vi "CheckInputFrequency.vi"(4 "Connection ID TB":refnum<k5>, 5 "ERROR IN":errorcluster, 6 "IP ADDRESS":string="192.168.0.2", 7 "TS1 / TS2":bool, 8 "Connection ID CC":refnum<k5>) -> (0 "ERROR OUT":errorcluster, 1 "Success":bool=TRUE, 3 "String":string)   [LabVIEW 2013]
panel:
  out "PROGRESS":i32(slide) scale=0.0..12.0
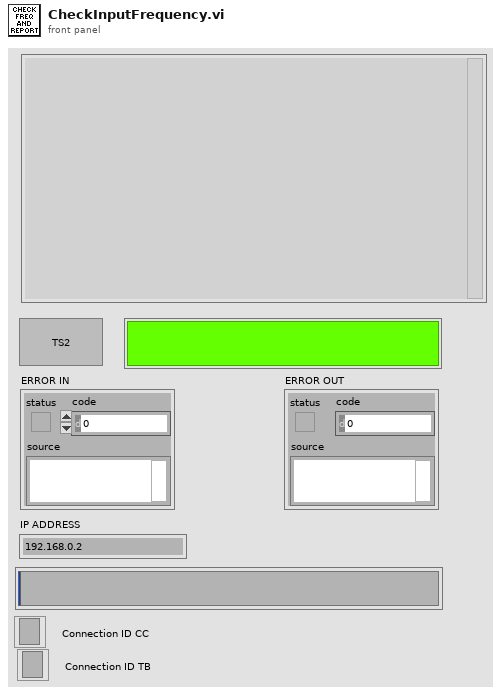
[diagram p1: front panel]
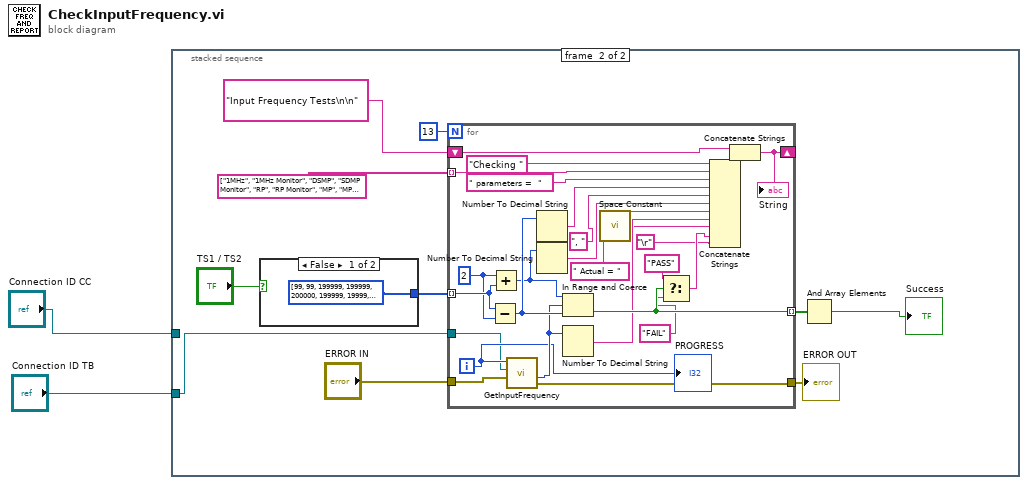
[diagram p0: block diagram]
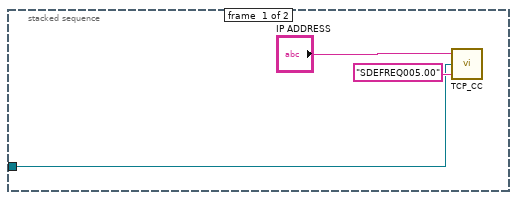
[diagram p2: hidden frame]
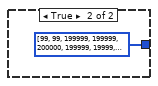
[diagram p3: hidden frame]
diagram:
  n1 = stacked-sequence {
    tunnel: "Connection ID CC" -> [w3 _]
    tunnel: "Connection ID TB" -> [_ w6]
    frame #0 {
      n2 = call "TCP_CC.vi"("COMMAND"="SDEFREQ005.00", "connection ID"=w3, "IP ADDRESS"="IP ADDRESS") -> ()  [unwired: 3 out]
    }
    frame #1 {
      n3 = case shown="False" "TS1 / TS2" {
        tunnel: [u32[] [99, 99, 199999, 199999, 200000, 199999, 19999, 19999, 1199999, 99999, 199999, 199999, 199999] ("Array") u32[] [99, 99, 199999, 199999, 200000, 199999, 19999, 19999, 1199999, 99999, 199999, 199999, 199999] ("Array")] -> w12
        frame False {
        }
        frame True {
        }
      }
      n4 = for {
        N: 13 -> [_]
        tunnel: "ERROR IN" -> [w43]
        tunnel: [w42] -> w14
        tunnel: w12 -> [w20] mode=indexing
        tunnel: [w37] -> w8 mode=indexing
        tunnel: string[] ["1MHz", "1MHz Monitor", "DSMP", "SDMP Monitor", "RP", "RP Monitor", "MP", "MP Monitor", "EEP 1.2", "EEP Monitor", "SMP DIFF", "SMP Monitor", "SMP OC"] -> [w31] mode=indexing
        shift-right: [w21] -> _
        shift-left: "Input Frequency Tests\n\n" -> [w33]
        tunnel: w6 -> [w18]
        i -> [w22]
        w19 = u32 2 ("x")
        n5 = Subtract(x=w20, y=w19) -> (x-y=w41:u32)
        n6 = Add(x=w19, y=w20) -> (x+y=w40:u32)
        n7 = call "GetInputFrequency.vi"("Signal Type Select"=w22, "Connection ID IN"=w18, "ERROR IN"=w43) -> ("DECIMAL"=w38:u32, "ERROR OUT"=w42:errorcluster)  [unwired: 2 in, 2 out]
        n8 = Number To Decimal String(number=w41) -> (decimal integer string=w29:string)  [unwired: 1 in]
        n9 = Number To Decimal String(number=w40) -> (decimal integer string=w39:string)  [unwired: 1 in]
        n10 = In Range and Coerce(upper limit=w40, x=w38, lower limit=w41) -> (In Range?=w37:bool)  [unwired: 1 out]
        n11 = Number To Decimal String(number=w38) -> (decimal integer string=w26:string)  [unwired: 1 in]
        n12 = call <vilib>:"Space Constant.vi"() -> ("String"=w25:string)
        n13 = Select(t="PASS", s=w37, f="FAIL") -> (s? t:f=w24:string)
        n14 = Concatenate Strings("Checking ", w31, " parameters =  ", w29, ", ", w39, " Actual = ", w26, w25, w24, "\r") -> (w34:string)
        n15 = Concatenate Strings(w33, w34) -> (w21:string)
        "String" <- w21
        "PROGRESS" <- w22
      }
      "ERROR OUT" <- w14
      n16 = And Array Elements(Boolean array=w8) -> (logical AND=→"Success":bool)
    }
  }
